vi "TCP Write to Connection.vi"(5 "Options":T1={"Ignore Timeout Error"=FALSE, "timeout ms (1000)"=1000}, 7 "error in":errorcluster, 8 "index":i32, 9 "Variant":variant, 10 "Meta data Name":string) -> (0 "error out":errorcluster)   [LabVIEW 2010]
doc: "This VI writes a package of data to the connection specified by \"index\". It also prepends a specified meta data ID to each packet. \n\nThis VI is responsible for flattening the desired data to a string before transmission."
uses:
  stm_TCP Write Options.ctl
  Connection Manager/TCP/TCP Connection Method.ctl
  NI STM.lvlib
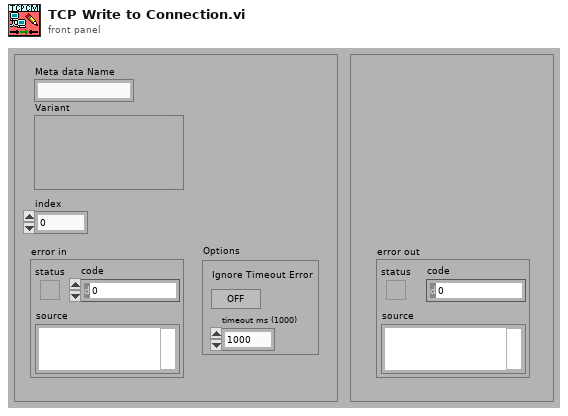
[diagram p1: front panel]
types:
  T1 = typedef "stm_TCP Write Options.ctl" = cluster{"Ignore Timeout Error":bool, "timeout ms (1000)":i32}
  T2 = typedef "NI STM.lvlib/TCP Connection Method.ctl" = enum16{"Initialize", "Add Connection", "Set Properties", "Get Connection(s)", "Remove Connection", "Remove All Connections", "Get Connection Count"}
  T3 = typedef "NI STM.lvlib/TCP Connection Info.ctl" = cluster{"connection ID":refnum<k5>, "Meta data":T4[]}
  T4 = typedef "NI STM.lvlib/MetaDataElement.ctl" = string
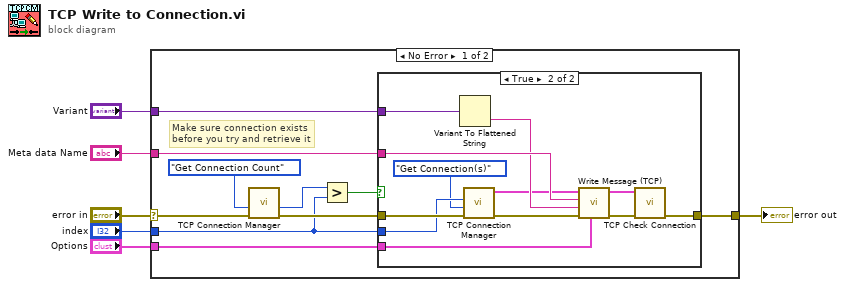
[diagram p0: block diagram]
diagram:
  n1 = case shown="No Error" "error in" {
    selector: "error in" -> [w12 w30]
    tunnel: "Variant" -> [w16 _]
    tunnel: "Meta data Name" -> [w15 _]
    tunnel: [w14 w30] -> w4
    tunnel: "index" -> [w9 _]
    tunnel: "Options" -> [w8 _]
    frame No Error {
      # "Make sure connection exists\nbefore you try and retrieve it"
      n2 = call "TCP Connection Manager.vi"("error in"=w12, "Method"=TCP_Connection_Method."Get Connection Count") -> ("error out"=w13:errorcluster, "Number of Connections"=w11:i32)  [unwired: 4 in, 4 out]
      n3 = Greater?(x=w11, y=w9) -> (0:w10:bool)
      n4 = case shown="True" w10 {
        tunnel: w13 -> [w17 w22]
        tunnel: [w17 w29] -> w14
        tunnel: w15 -> [_ w27]
        tunnel: w16 -> [_ w26]
        tunnel: w9 -> [_ w20]
        tunnel: w8 -> [_ w19]
        frame False {
        }
        frame True {
          n5 = Variant To Flattened String(Variant=w26) -> (data string=w25:string)  [unwired: 1 out]
          n6 = call "TCP Connection Manager.vi"("error in"=w22, "Method"=TCP_Connection_Method."Get Connection(s)", "Index"=w20) -> ("error out"=w21:errorcluster, "Connection Out"=w23:T3)  [unwired: 3 in, 4 out]
          n7 = call "Write Message (TCP).vi"("Options"=w19, "error in"=w21, "Data"=w25, "Name"=w27, "Connection Info"=w23) -> ("error out"=w24:errorcluster, "Connection Info Out"=w28:T3)  [unwired: 5 in]
          n8 = call "TCP Check Connection.vi"("error in"=w24, "Connection In"=w28) -> ("error out"=w29:errorcluster)  [unwired: 7 in, 2 out]
        }
      }
    }
    frame Error {
    }
  }
  "error out" <- w4
